vi "Obtain and Save.vi"(8 "error in (no error)":errorcluster, 11 "EventLog in":refnum<class "EventLog.lvclass">) -> (0 "error out":errorcluster, 3 "EventLog out":refnum<class "EventLog.lvclass">)   [LabVIEW 2019, in "EventLog.lvlib" / "EventLog.lvclass"]
uses:
  EventLog.lvclass
  LogsAbstract/LogsAbstract.lvclass
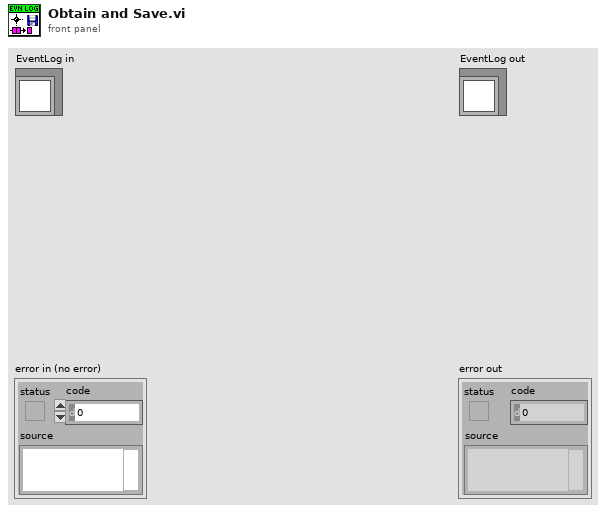
[diagram p1: front panel]
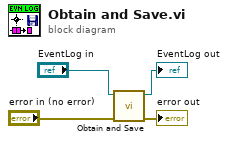
[diagram p0: block diagram]
diagram:
  n1 = call-parent "Obtain and Save.vi"("error in (no error)"="error in (no error)", "LogsAbstract in"="EventLog in") -> ("error out"=→"error out":errorcluster, "LogsAbstract out"=→"EventLog out":refnum<class "EventLog.lvclass">)  [unwired: 8 in]
